vi "set transfer info.vi"(8 "error in (no error)":errorcluster, 9 "transfer info":T1, 10 "id":string, 11 "DSFConfiguration in":refnum<class "DSFConfiguration.lvclass">) -> (0 "error out":errorcluster, 3 "DSFConfiguration out":refnum<class "DSFConfiguration.lvclass">)   [LabVIEW 2017, in "DSFConfiguration.lvclass"]
uses:
  DSFConfiguration.lvclass
  Controls/dsf configuration file/1.0.0/dsf transfer.ctl
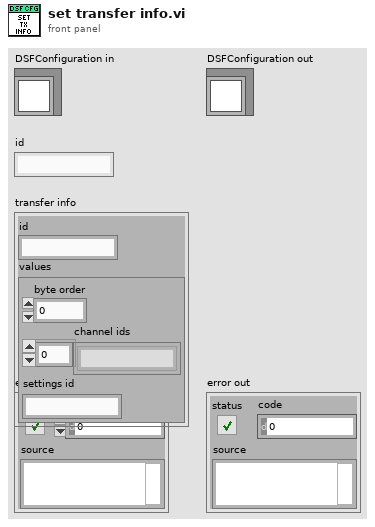
[diagram p1: front panel]
types:
  T1 = typedef "dsf configuration file v1.0.0.lvlib/dsf transfer.ctl" = cluster{"id":string, "values":cluster{"byte order":i32, "channel ids":string[], "settings id":string}}
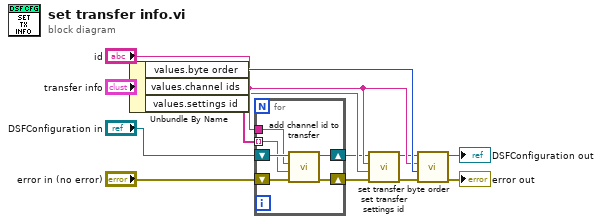
[diagram p0: block diagram]
diagram:
  n1 = Unbundle By Name("transfer info") -> ("values.byte order"=w13:i32, "values.channel ids"=w7:string[], "values.settings id"=w8:string)
  n2 = for {
    shift-right: [w18] -> w5
    shift-left: "error in (no error)" -> [w19]
    shift-right: [w16] -> w6
    shift-left: "DSFConfiguration in" -> [w17]
    tunnel: "id" -> [w15]
    tunnel: w7 -> [w14] mode=indexing
    n3 = call "add channel id to transfer.vi"("error in (no error)"=w19, "channel id"=w14, "id"=w15, "DSFConfiguration in"=w17) -> ("error out"=w18:errorcluster, "DSFConfiguration out"=w16:refnum<class "DSFConfiguration.lvclass">)  [unwired: 6 in]
  }
  n4 = call "set transfer settings id.vi"("error in (no error)"=w5, "settings id"=w8, "id"="id", "DSFConfiguration in"=w6) -> ("error out"=w4:errorcluster, "DSFConfiguration out"=w10:refnum<class "DSFConfiguration.lvclass">)  [unwired: 6 in]
  n5 = call "set transfer byte order.vi"("error in (no error)"=w4, "byte order"=w13, "id"="id", "DSFConfiguration in"=w10) -> ("error out"=→"error out":errorcluster, "DSFConfiguration out"=→"DSFConfiguration out":refnum<class "DSFConfiguration.lvclass">)  [unwired: 6 in]
